vi "_PC_Pub_FM readProperty.vi"(7 "readEvent":T1, 8 "error in (no error)":errorcluster, 10 "timeStamp":string, 11 "FM in":refnum<class "FM.lvclass">) -> (0 "error out":errorcluster, 2 "outputArr":string[][](array[string]), 3 "FM out":refnum<class "FM.lvclass">)   [LabVIEW 2018, in "FM.lvclass"]
uses:
  FM.lvclass
  ctl/_PC_Pub_FM fileReadFuncEnum.ctl
  FM.lvclass/FM.ctl
  TDMSAdv.lvclass
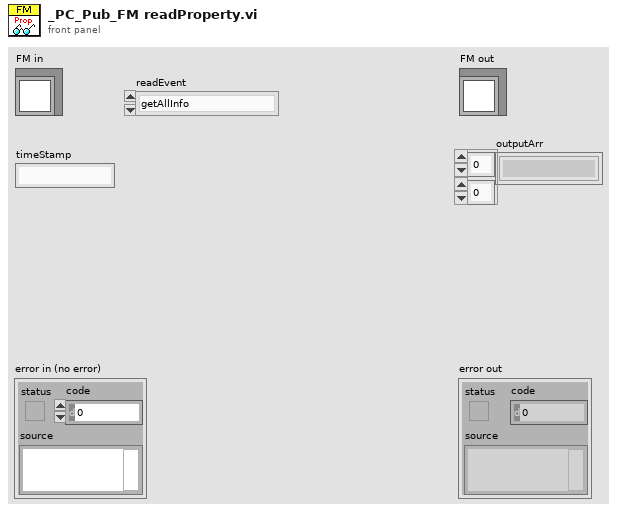
[diagram p1: front panel]
types:
  T1 = typedef "_PC_Pub_FM fileReadFuncEnum.ctl" = enum16{"getAllInfo", "getChromatogram", "getDataItems", "getTimeStamp", "getIdxData", "getIonization", "getRemark", "getAttrFormat"}
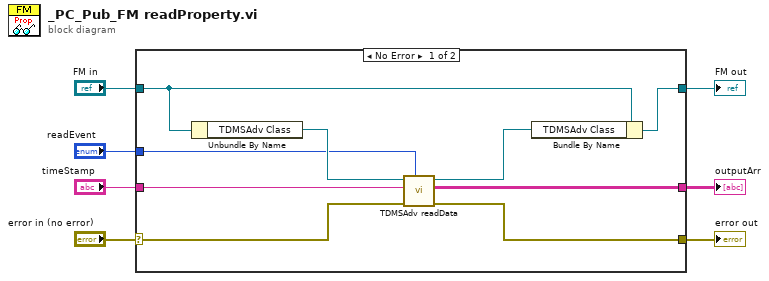
[diagram p0: block diagram]
diagram:
  n1 = case shown="No Error" "error in (no error)" {
    selector: "error in (no error)" -> [w11 w18]
    tunnel: [w10 w18] -> w6
    tunnel: [w13 w17] -> w4
    tunnel: "FM in" -> [w15 w17]
    tunnel: "readEvent" -> [w12 _]
    tunnel: [w9 _] -> w2
    tunnel: "timeStamp" -> [w8 _]
    frame No Error {
      n2 = Unbundle By Name(w15) -> ("TDMSAdv Class"=w16:refnum<class "TDMSAdv.lvclass">)
      n3 = call "TDMSAdv readData.vi"("readEvent"=w12, "error in (no error)"=w11, "timeStamp"=w8, "TDMSAdv in"=w16) -> ("error out"=w10:errorcluster, "outputArr"=w9:string[][], "TDMSAdv out"=w14:refnum<class "TDMSAdv.lvclass">)  [unwired: 4 in, 1 out]
      n4 = Bundle By Name(cluster=w15, "TDMSAdv Class"=w14) -> (w13:refnum<class "FM.lvclass">)
    }
    frame Error {
    }
  }
  "error out" <- w6
  "FM out" <- w4
  "outputArr" <- w2
